vi "Subsystem 10.vi"(10 "v1":dbl(slide)=2.9591836734693877 scale=0.0..5.0, 11 "v2":dbl(slide)=3.010204081632653 scale=0.0..5.0) -> (2 "H1":dbl, 3 "H2":dbl)   [LabVIEW 2015]
uses:
  <vilib>/Simulation/Implementation/Shared/SIMSCR Execution Mode.ctl
  <vilib>/Simulation/Scripting/Companion Diagram/SimConfigNode/SimParams.ctl
  <vilib>/Simulation/Scripting/Companion Diagram/SimConfigNode/_simSolvers.ctl
  <vilib>/Simulation/Param Hierarchy/Typedefs/SIMPH Param Control Actions.ctl
  <vilib>/Simulation/Implementation/Shared/SIM limit type.ctl
  <vilib>/Simulation/Implementation/Shared/NILVSim_ParamChanged.vi
  <vilib>/Simulation/Implementation/Shared/NILVSIM_BeginStep.vi
  <vilib>/Simulation/ContinuousLinear/Implementation/NILVSim Integrator new.llb/SIM Integrator distributor (scalar).vi
  <vilib>/Simulation/Nonlinear/Implementation/NILVSim Saturation.llb/SIM Saturation (scalar).vi
  <vilib>/Simulation/ContinuousLinear/Implementation/NILVSim Integrator new.llb/SIM Integrator collector (scalar).vi
  <vilib>/Simulation/Implementation/Shared/NILVSim_Manager.vi
  <vilib>/Utility/error.llb/Clear Errors.vi
  <vilib>/Simulation/Implementation/Shared/NILVSim_FinalizeModel.vi
  <vilib>/Simulation/Implementation/Shared/SIM Unbundle Sim Info.vi
  <vilib>/Simulation/Implementation/Shared/SIMSH Read Queue.vi
  <vilib>/Simulation/Implementation/Shared/NILVSim_Initialize.vi
  <vilib>/Simulation/Utility/Implementation/NILVSim Get Time and IsAcceptedStep.vi
  <vilib>/Simulation/Implementation/Shared/NILVSim_GetModelError.vi
  <vilib>/Simulation/Implementation/Shared/SIM SimErrorHandler.vi
  <vilib>/Simulation/Implementation/Shared/SIM Bundle Sim Info.vi
  <vilib>/Simulation/Scripting/Companion Diagram/SimConfigNode/SimDog.xnode
  <vilib>/Simulation/Implementation/XNodeFramework/SimXNode/SimX.xnode
  <vilib>/Simulation/ContinuousLinear/Implementation/NILVSim Integrator new.llb/SIM Integrator (scalar).vi
  <vilib>/Simulation/Implementation/Shared/NI_SIM_Implementation.lvlib
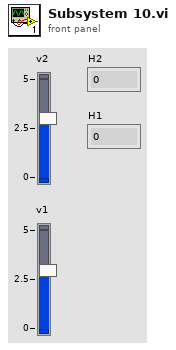
[diagram p1: front panel]
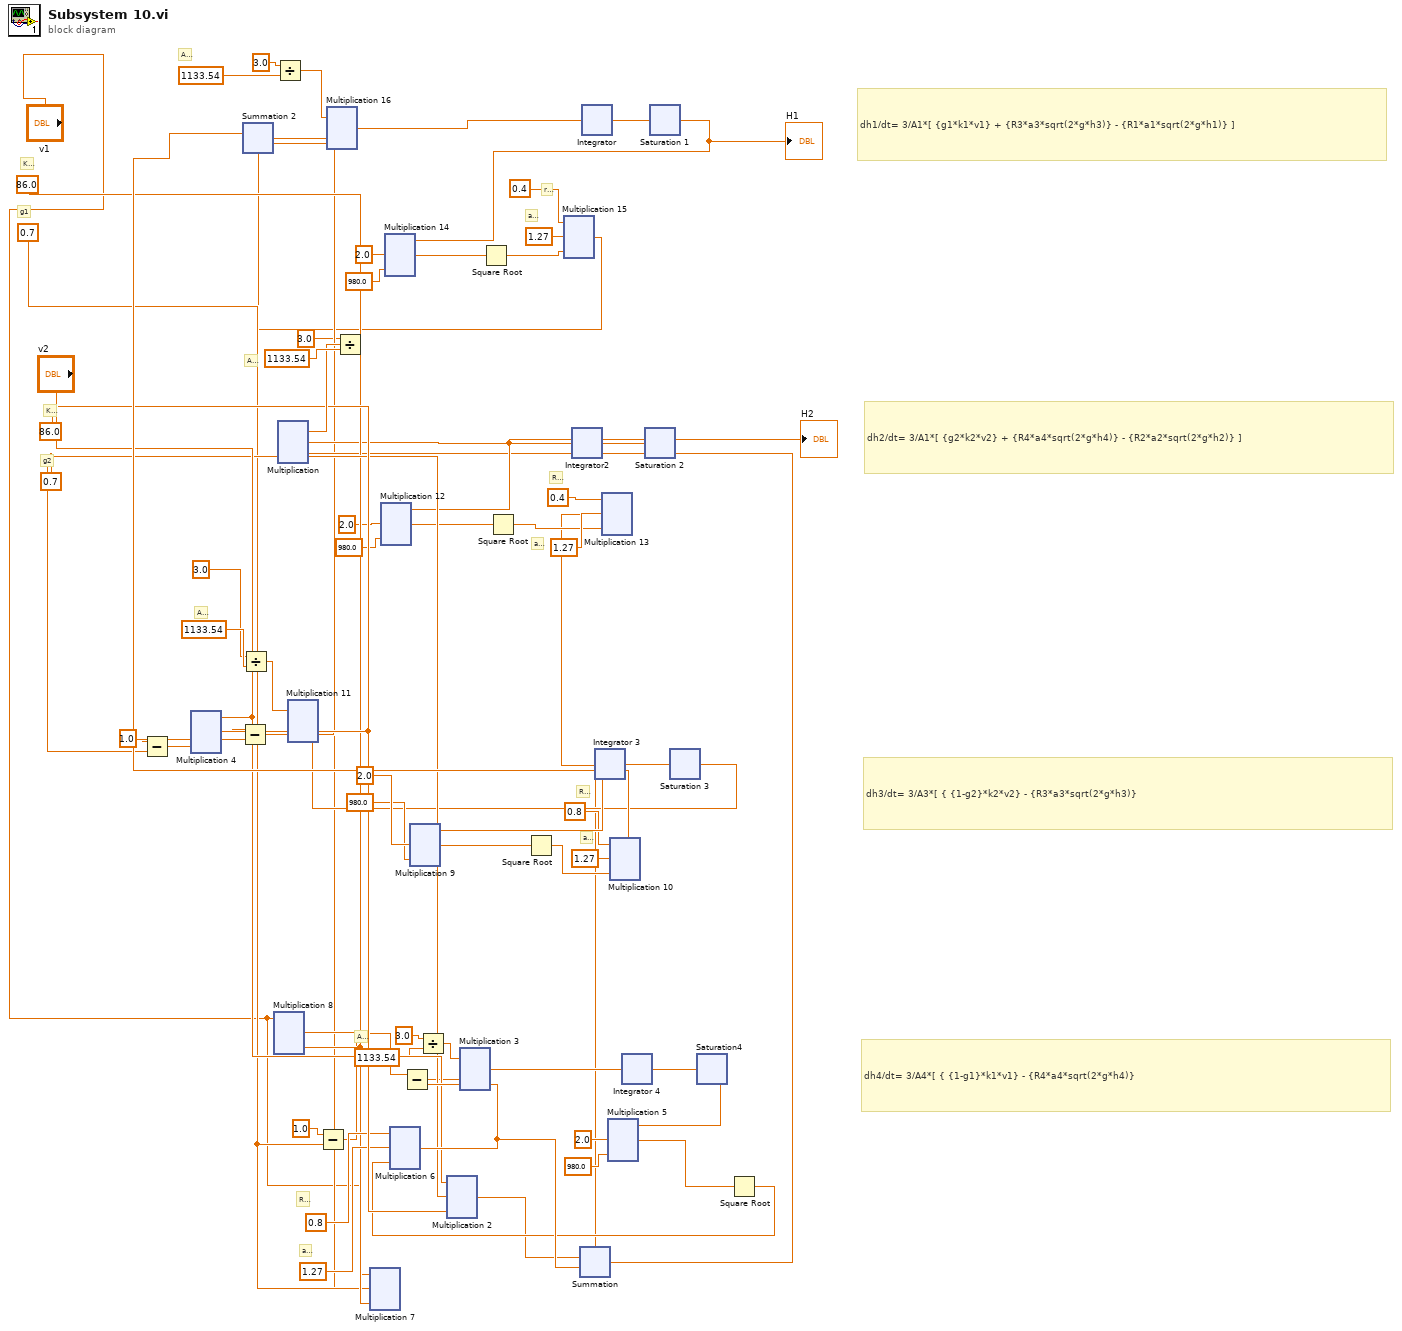
[diagram p0: block diagram]
diagram:
  w48 = 86.0 ("K 2")
  w46 = 0.7 ("g2")
  w63 = 86.0 ("K1")
  w61 = 0.7 ("g1")
  # "dh4/dt= 3/A4*[ { {1-g1}*k1*v1} - {R4*a4*sqrt(2*g*h4)}"
  # "dh3/dt= 3/A3*[ { {1-g2}*k2*v2} - {R3*a3*sqrt(2*g*h3)}"
  # "dh2/dt= 3/A1*[ {g2*k2*v2} + {R4*a4*sqrt(2*g*h4)} - {R2*a2*sqrt(2*g*h2)} ]"
  # "dh1/dt= 3/A1*[ {g1*k1*v1} + {R3*a3*sqrt(2*g*h3)} - {R1*a1*sqrt(2*g*h1)} ]"
  # "R2"
  # "a3"
  # "R3"
  # "A3"
  # "K1"
  # "g1"
  # "a1"
  # "r1"
  # "A1"
  # "a4"
  # "R4"
  # "A4"
  # "a2"
  # "A2"
  # "K2"
  # "g2"
  n1 = Subtract(x=1.0 ("x 5"), y=w61) -> (x-y=w60:dbl)
  n2 = xnode "Multiplication 4"("Operand1"="v2", "Operand2"=w63, "Operand3"=w60) -> ("Result"=w8:dbl)
  n3 = Divide ("Divide 3")(x=3.0 ("x 7"), y=1133.54 ("A3")) -> (x/y=w35:dbl)
  n4 = Divide ("Divide 4")(x=3.0 ("x 8"), y=1133.54 ("A 2")) -> (x/y=w11:dbl)
  n5 = Subtract ("Subtract 3")(x=1.0 ("x 6"), y=w46) -> (x-y=w45:dbl)
  n6 = xnode "Multiplication 8"("Operand1"="v1", "Operand2"=w45, "Operand3"=w48) -> ("Result"=w7:dbl)
  n7 = Divide(x=3.0 ("x 3"), y=1133.54 ("A1")) -> (x/y=w66:dbl)
  n8 = xnode "Multiplication 7"("Operand1"="v1", "Operand2"=w46, "Operand3"=w48) -> ("Result"=w20:dbl)
  n9 = Divide ("Divide 2")(x=3.0 ("x 4"), y=1133.54 ("A4")) -> (x/y=w64:dbl)
  n10 = xnode "Multiplication 2"("Operand1"="v2", "Operand2"=w61, "Operand3"=w63) -> ("Result"=w32:dbl)
  n11 = Subtract ("Subtract 4")(x=w8, y=w69) -> (x-y=w34:dbl)
  n12 = xnode "Multiplication 11"("Operand1"=w35, "Operand2"=w34) -> ("Result"=w33:dbl)
  n13 = xnode "Integrator 3"("input"=w33) -> ("output"=w44:dbl)  [unwired: 9 in, 2 out]
  n14 = xnode "Saturation 3"("input"=w44) -> ("output"=w43:dbl)  [unwired: 4 in]
  n15 = xnode "Multiplication 9"("Operand1"=w43, "Operand2"=2.0, "Operand3"=980.0 ("Operand3 2")) -> ("Result"=w40:dbl)
  n16 = Square Root ("Square Root 2")(x=w40) -> (sqrt(x)=w37:dbl)
  n17 = xnode "Multiplication 10"("Operand1"=0.8 ("R3"), "Operand2"=1.27 ("a3"), "Operand3"=w37) -> ("Result"=w69:dbl)
  n18 = xnode "Summation 2"("Operand1"=w69, "Operand2"=w20, "Operand3"=w14) -> ("Result"=w10:dbl)
  n19 = xnode "Multiplication 16"("Operand1"=w11, "Operand2"=w10) -> ("Result"=w9:dbl)
  n20 = xnode "Integrator"("input"=w9) -> ("output"=w19:dbl)  [unwired: 9 in, 2 out]
  n21 = xnode "Saturation 1"("input"=w19) -> ("output"=w3:dbl)  [unwired: 4 in]
  "H1" <- w3
  n22 = xnode "Multiplication 14"("Operand1"=w3, "Operand2"=2.0 ("Operand2 3"), "Operand3"=980.0 ("Operand3 4")) -> ("Result"=w6:dbl)
  n23 = Square Root ("Square Root 4")(x=w6) -> (sqrt(x)=w5:dbl)
  n24 = xnode "Multiplication 15"("Operand1"=0.4 ("R2"), "Operand2"=1.27 ("a 2"), "Operand3"=w5) -> ("Result"=w14:dbl)
  n25 = xnode "Multiplication"("Operand1"=w66, "Operand2"=w22) -> ("Result"=w21:dbl)
  n26 = xnode "Integrator2"("input"=w21) -> ("output"=w31:dbl)  [unwired: 9 in, 2 out]
  n27 = xnode "Saturation 2"("input"=w31) -> ("output"=w30:dbl)  [unwired: 4 in]
  "H2" <- w30
  n28 = xnode "Multiplication 12"("Operand1"=w30, "Operand2"=2.0 ("Operand2 2"), "Operand3"=980.0 ("Operand3 3")) -> ("Result"=w27:dbl)
  n29 = Square Root ("Square Root 3")(x=w27) -> (sqrt(x)=w24:dbl)
  n30 = xnode "Multiplication 13"("Operand1"=0.4 ("R1"), "Operand2"=1.27 ("a1"), "Operand3"=w24) -> ("Result"=w23:dbl)
  n31 = xnode "Multiplication 6"("Operand1"=0.8 ("R4"), "Operand2"=1.27 ("a 4"), "Operand3"=w52) -> ("Result"=w70:dbl)
  n32 = Subtract ("Subtract 2")(x=w7, y=w70) -> (x-y=w50:dbl)
  n33 = xnode "Multiplication 3"("Operand1"=w64, "Operand2"=w50) -> ("Result"=w49:dbl)
  n34 = xnode "Summation"("Operand1"=w32, "Operand2"=w70, "Operand3"=w23) -> ("Result"=w22:dbl)
  n35 = xnode "Integrator 4"("input"=w49) -> ("output"=w59:dbl)  [unwired: 9 in, 2 out]
  n36 = xnode "Saturation4"("input"=w59) -> ("output"=w58:dbl)  [unwired: 4 in]
  n37 = xnode "Multiplication 5"("Operand1"=w58, "Operand2"=2.0 ("y"), "Operand3"=980.0) -> ("Result"=w55:dbl)
  n38 = Square Root(x=w55) -> (sqrt(x)=w52:dbl)
